vi "Fit VI window to Content.vi"(4 "error in (no error)":errorcluster, 6 "border spacing (2 px)":i32=2, 7 "VI Ref":refnum<vi>) -> (0 "error out":errorcluster, 3 "dup VI Ref":refnum<vi>)   [LabVIEW 2017, in "csm-ui-support.lvlib"]
doc: "This utility will fit (resize and center) a VI (defined by the \"VI Ref\" input) about the all of the Front Panel object. It will add a border defined by border spacing in units of pixels. If no VI Reference is passed in, it will operate on the calling VI."
uses:
  csm-ui-support.lvlib
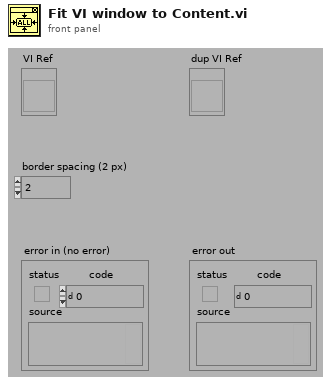
[diagram p1: front panel]
types:
  T1 = typedef "LVRectTypeDef.ctl" = cluster{"Left":i16, "Top":i16, "Right":i16, "Bottom":i16}
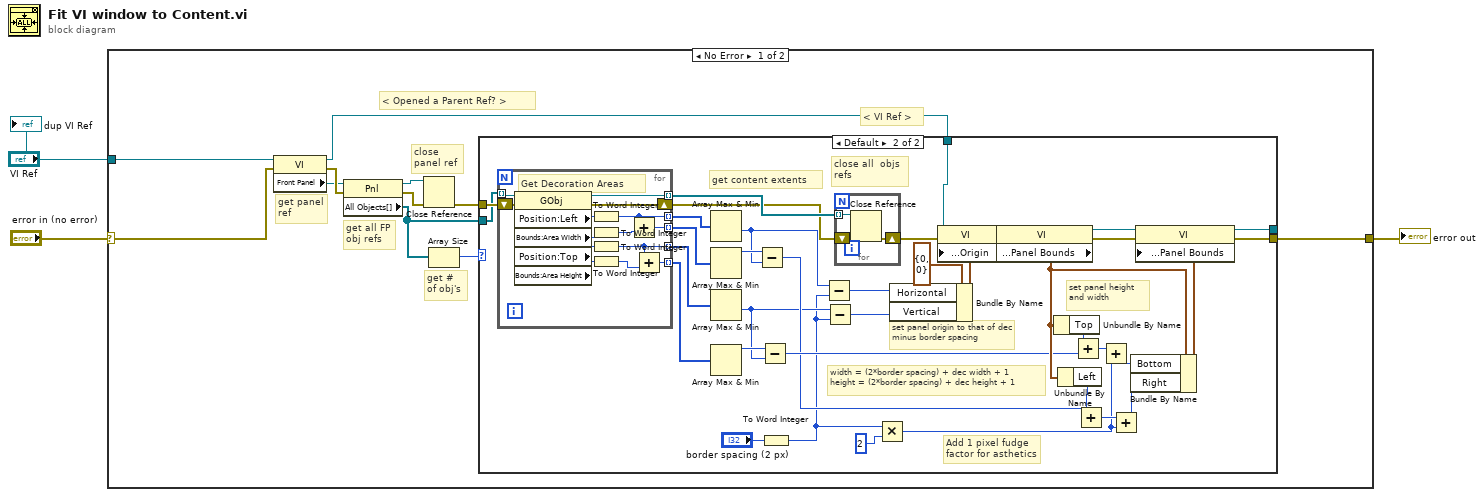
[diagram p0: block diagram]
diagram:
  n1 = case shown="No Error" "error in (no error)" {
    selector: "error in (no error)" -> [w5 w72]
    tunnel: [w8 w72] -> w3
    tunnel: "VI Ref" -> [w4 _]
    frame No Error {
      # "< Opened a Parent Ref? >"
      # "get # of obj's"
      # "get panel ref"
      # "get all FP obj refs"
      # "close panel ref"
      # "< VI Ref >"
      n2 = property on="Property Node" class="VI"(reference=w4, error in=w5) -> (reference out=w14:refnum<vi>, error out=w12:errorcluster, "Front Panel"=w10:refnum<vi>)
      n3 = property on="Property Node" class="Pnl"(reference=w10, error in=w12) -> (reference out=w13:refnum<vi>, error out=w11:errorcluster, "All Objects[]"=w7:refnum<vi>[])
      n4 = Close Reference(reference=w13, error in (no error)=w11) -> (error out=w9:errorcluster)
      n5 = Array Size(array=w7) -> (size(s)=w6:i32)
      n6 = case shown="Default" w6 {
        tunnel: w14 -> [w16 w52]
        tunnel: w9 -> [w15 w39]
        tunnel: [w15 w34] -> w8
        tunnel: [w16 w33] -> _
        tunnel: w7 -> [_ w32]
        frame 0 {
          # "do nothing if no objects"
        }
        frame Default {
          # "width = (2*border spacing) + dec width + 1\nheight = (2*border spacing) + dec height + 1"
          # "set panel height and width"
          # "set panel origin to that of dec minus border spacing"
          # "close all  objs refs"
          # "get content extents"
          # "Add 1 pixel fudge factor for asthetics"
          n7 = for {
            tunnel: w32 -> [w71] mode=indexing
            shift-right: [w69] -> w19
            shift-left: w39 -> [w70]
            tunnel: [w68] -> w20 mode=indexing
            tunnel: [w64] -> w30 mode=indexing
            tunnel: [w66] -> w29 mode=indexing
            tunnel: [w60] -> w28 mode=indexing
            tunnel: [w65] -> w27 mode=indexing
            # "Get Decoration Areas"
            n8 = property class="GObj"(reference=w71, error in=w70) -> (reference out=w68:refnum<vi>, error out=w69:errorcluster, "Position:Left"=w67:i32, "Bounds:Area Width"=w63:u32, "Position:Top"=w61:i32, "Bounds:Area Height"=w59:u32)
            n9 = To Word Integer(number=w67) -> (16bit integer=w64:i16)
            n10 = To Word Integer(number=w63) -> (16bit integer=w62:i16)
            n11 = To Word Integer(number=w61) -> (16bit integer=w60:i16)
            n12 = To Word Integer(number=w59) -> (16bit integer=w58:i16)
            n13 = Add(x=w64, y=w62) -> (x+y=w66:i16)
            n14 = Add(x=w60, y=w58) -> (x+y=w65:i16)
          }
          n15 = Array Max & Min(array=w30) -> (min value=w21:i16)  [unwired: 3 out]
          n16 = Array Max & Min(array=w29) -> (max value=w24:i16)  [unwired: 3 out]
          n17 = Array Max & Min(array=w28) -> (min value=w22:i16)  [unwired: 3 out]
          n18 = Array Max & Min(array=w27) -> (max value=w26:i16)  [unwired: 3 out]
          n19 = Subtract(x=w24, y=w21) -> (x-y=w23:i16)
          n20 = Subtract(x=w26, y=w22) -> (x-y=w25:i16)
          n21 = To Word Integer(number="border spacing (2 px)") -> (16bit integer=w17:i16)
          n22 = Subtract(x=w21, y=w17) -> (x-y=w42:i16)
          n23 = Subtract(x=w22, y=w17) -> (x-y=w43:i16)
          n24 = for {
            tunnel: w20 -> [w57] mode=indexing
            shift-right: [w55] -> w18
            shift-left: w19 -> [w56]
            n25 = Close Reference(reference=w57, error in (no error)=w56) -> (error out=w55:errorcluster)
          }
          n26 = Multiply(x=w17, y=i16 2) -> (x*y=w31:i16)
          n27 = Bundle By Name(cluster=cluster{"Horizontal":i16, "Vertical":i16} {"Horizontal"=0, "Vertical"=0} ("Front Panel Window:Origin"), "Horizontal"=w42, "Vertical"=w43) -> (w40:cluster{"Horizontal":i16, "Vertical":i16})
          n28 = property on="Property Node" class="VI"(reference=w52, error in=w18, "Front Panel Window:Origin"=w40) -> (reference out=w53:refnum<vi>, error out=w36:errorcluster)
          n29 = property on="Property Node" class="VI"(reference=w53, error in=w36) -> (reference out=w54:refnum<vi>, error out=w35:errorcluster, "Front Panel Window:Panel Bounds"=w44:T1)
          n30 = Unbundle By Name(w44) -> ("Top"=w45:i16)
          n31 = Unbundle By Name(w44) -> ("Left"=w46:i16)
          n32 = Add(x=w45, y=w25) -> (x+y=w50:i16)
          n33 = Add(x=w46, y=w23) -> (x+y=w48:i16)
          n34 = Add(x=w50, y=w31) -> (x+y=w51:i16)
          n35 = Add(x=w48, y=w31) -> (x+y=w49:i16)
          n36 = Bundle By Name(cluster=w44, "Bottom"=w51, "Right"=w49) -> (w47:T1)
          n37 = property on="Property Node" class="VI"(reference=w54, error in=w35, "Front Panel Window:Panel Bounds"=w47) -> (reference out=w33:refnum<vi>, error out=w34:errorcluster)
        }
      }
    }
    frame Error {
    }
  }
  "error out" <- w3
  "dup VI Ref" <- "VI Ref"
